vi "选中背景色.vi"(8 "错误输入（无错误）":errorcluster, 11 "引用":refnum<k24>) -> (0 "错误输出":errorcluster, 3 "引用输出":refnum<k24>)   [LabVIEW 2018]
uses:
  ScintillaNET.dll
  System.Drawing
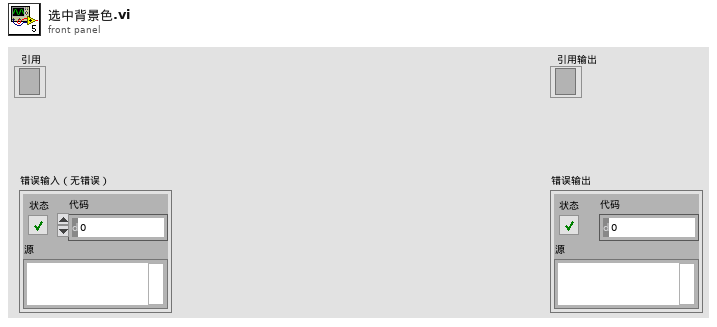
[diagram p1: front panel]
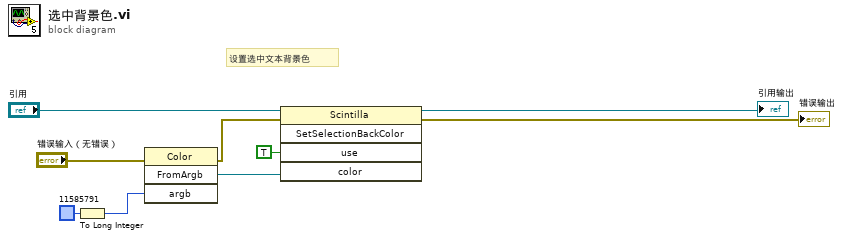
[diagram p0: block diagram]
diagram:
  # "设置选中文本背景色"
  n1 = To Long Integer(number=u32 11585791) -> (32bit integer=w7:i32)
  n2 = invoke class="Color" method="FromArgb"(error in="错误输入（无错误）", "argb"=w7) -> (error out=w4:errorcluster, "FromArgb"=w1:refnum<k24>)  [unwired: 2 in, 2 out]
  n3 = invoke class="Scintilla" method="SetSelectionBackColor"(reference="引用", error in=w4, "use"=TRUE, "color"=w1) -> (reference out=→"引用输出":refnum<k24>, error out=→"错误输出":errorcluster)  [unwired: 1 in, 3 out]
